vi "L15.vi"() -> ()   [LabVIEW 2012]
panel:
  out "Array":i64[][](array[numeric])
  out "max value":i64
  out "Intensity Graph":i64[][](graph)
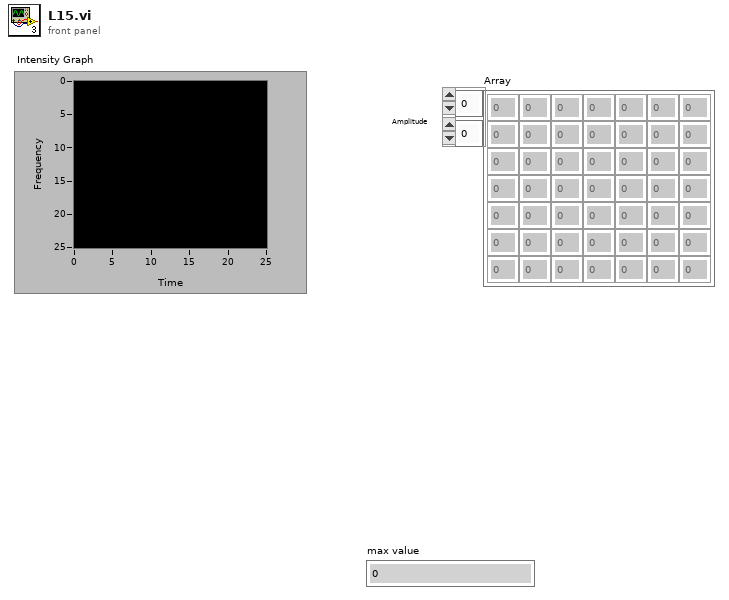
[diagram p1: front panel]
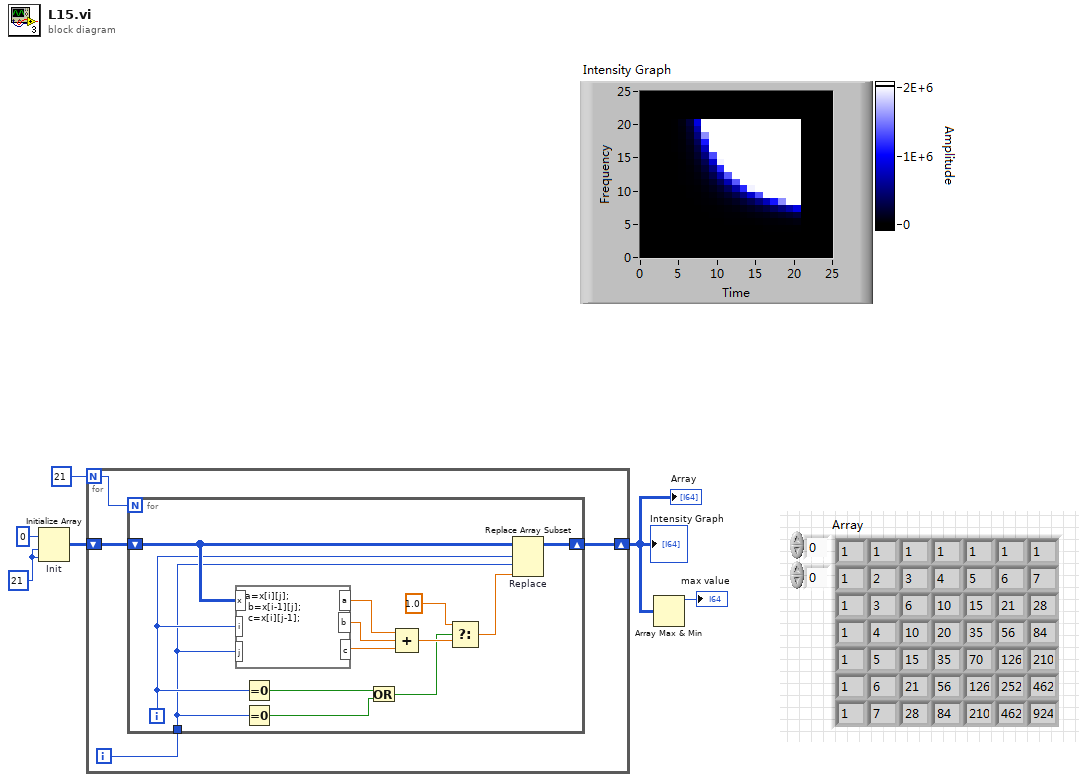
[diagram p0: block diagram]
diagram:
  w4 = 21 ("dimension size")
  n1 = Initialize Array "Init"(i64 0 ("element"), w4, w4) -> (w3:i64[][])
  n2 = for {
    N: 21 -> [w10]
    shift-right: [w7] -> w1
    shift-left: w3 -> [w9]
    i -> [w8]
    n3 = for {
      N: w10 -> [_]
      shift-right: [w17] -> w7
      shift-left: w9 -> [w16]
      tunnel: w8 -> [w14]
      i -> [w15]
      n4 = formula code="a=x[i][j];\n b=x[i-1][j];\n c=x[i][j-1];"("x"=w16, "i"=w15, "j"=w14) -> ("a"=w13:dbl, "b"=w12:dbl, "c"=w11:dbl)
      n5 = Equal To 0?(x=w15) -> (x = 0?=w23:bool)
      n6 = Equal To 0?(x=w14) -> (x = 0?=w22:bool)
      n7 = Or(x=w23, y=w22) -> (x .or. y?=w20:bool)
      n8 = Compound Arithmetic op=ADD(w13, w12, w11) -> (w21:dbl)
      n9 = Select(t=1.0 ("new element/subarray"), s=w20, f=w21) -> (s? t:f=w18:dbl)
      n10 = Replace Array Subset "Replace"(array=w16, new element=w18, index (row)=w15, index (col)=w14) -> (w17:i64[][])
    }
  }
  "Intensity Graph" <- w1
  "Array" <- w1
  n11 = Array Max & Min(array=w1) -> (max value=→"max value":i64)  [unwired: 3 out]
